vi "Read Control Experiment.json.vi"(8 "error in (no error)":errorcluster, 10 "file (use dialog)":path, 11 "SweepControl in":refnum<class "SweepControl.lvclass">) -> (0 "error out":errorcluster, 2 "output cluster":T1, 3 "SweepControl out":refnum<class "SweepControl.lvclass">)   [LabVIEW 2016, in "Control Experiment SM.lvclass"]
uses:
  Control Experiment SM.lvclass
  SweepControl/SweepControl.lvclass
  Typedefs/Control Experiment JSON--cluster.ctl
  <vilib>/addons/_JKI.lib/Serialization/JSON/JKI JSON Serialization.lvlib
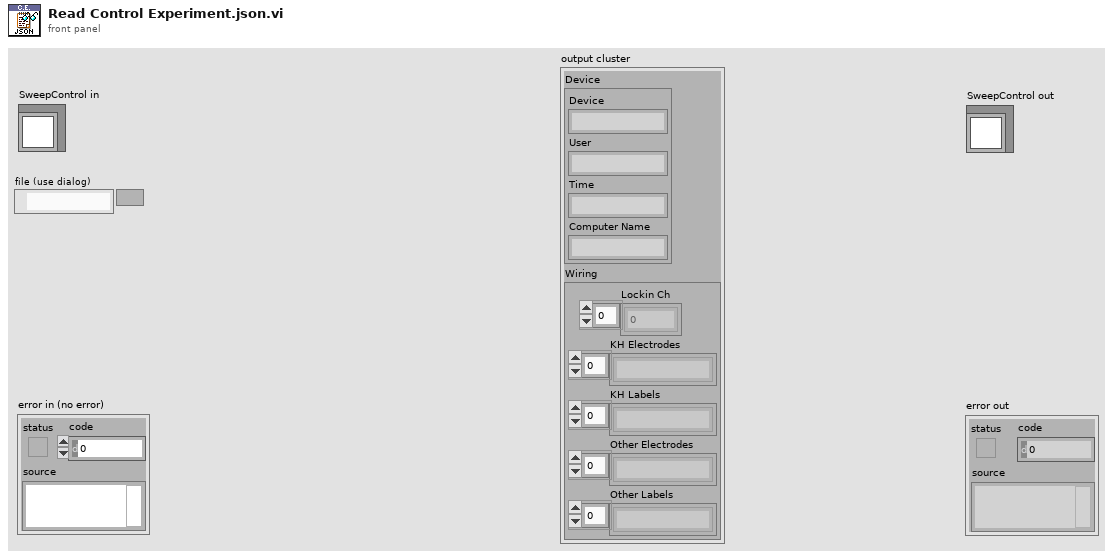
[diagram p1: front panel]
types:
  T1 = typedef "Control Experiment SM.lvclass/Control Experiment JSON--cluster.ctl" = cluster{"Device":cluster{"Device":string, "User":string, "Time":string, "Computer Name":string}, "Wiring":cluster{"Lockin Ch":u32[], "KH Electrodes":string[], "KH Labels":string[], "Other Electrodes":string[], "Other Labels":string[]}}
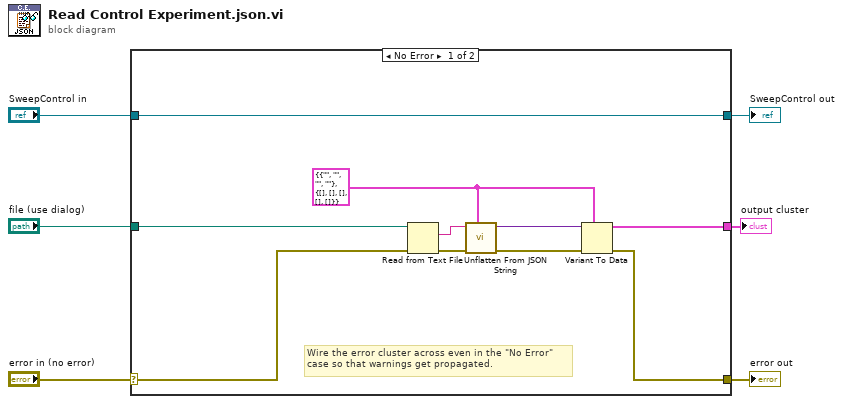
[diagram p0: block diagram]
diagram:
  n1 = case shown="No Error" "error in (no error)" {
    selector: "error in (no error)" -> [w13 w18]
    tunnel: [w11 w18] -> w5
    tunnel: [w16 w17] -> w3
    tunnel: "SweepControl in" -> [w16 w17]
    tunnel: "file (use dialog)" -> [w9 _]
    tunnel: [w8 _] -> w1
    frame No Error {
      w7 = T1 {"Device"={"Device"="", "User"="", "Time"="", "Computer Name"=""}, "Wiring"={"Lockin Ch"=[], "KH Electrodes"=[], "KH Labels"=[], "Other Electrodes"=[], "Other Labels"=[]}} ("output cluster")
      # "Wire the error cluster across even in the \"No Error\"\ncase so that warnings get propagated."
      n2 = Read from Text File(file (use dialog)=w9, error in=w13) -> (text=w14:string, error out=w15:errorcluster)  [unwired: 2 in, 2 out]
      n3 = call <vilib>:"Unflatten From JSON String.vi"("Type and Defaults"=w7, "error in (no error)"=w15, "JSON String"=w14) -> ("error out"=w12:errorcluster, "Variant"=w10:variant)  [unwired: 7 in]
      n4 = Variant To Data(error in=w12, type=w7, Variant=w10) -> (data=w8:T1, error out=w11:errorcluster)
    }
    frame Error {
    }
  }
  "error out" <- w5
  "SweepControl out" <- w3
  "output cluster" <- w1
